vi "Main Window.vi"() -> ()   [LabVIEW 2015]
uses:
  Control Button/Exit.ctl
  Control Button/login.ctl
  Control Button/Logout.ctl
  Control Button/setting.ctl
  Control Button/report.ctl
  Control Button/Manual.ctl
  Control Button/Start.ctl
  Enqueue/Main window Seq/Test selection_1.ctl
  Enqueue/Main window Seq/Test seq_1.ctl
  Galobal variable_TI.vi
  Project Setup/Globle Variable/GR_Servo.vi
panel:
  out "Boolean 3":bool
  out "Company Name  2":string
  out "Boolean 2":bool
  out "Error 2":bool
  out "Error":bool
  out "User Name":string
  out "error out":errorcluster
  out "x = y?":bool
  out "Company Name":string
  in  "Sign In":T1
  out "Boolean":bool
  in  "Dashbord":T6
  in  "Login Window":T8 {"User Name" items=["admin", "mmum", "a", "AJAY Kumar", "", "", "", "", "", "", "", "", "", "", "", "", "", "", "", "", "", "", "", "", "", "", "", "", "", "", "", ""]}
  in  "Exit":T9
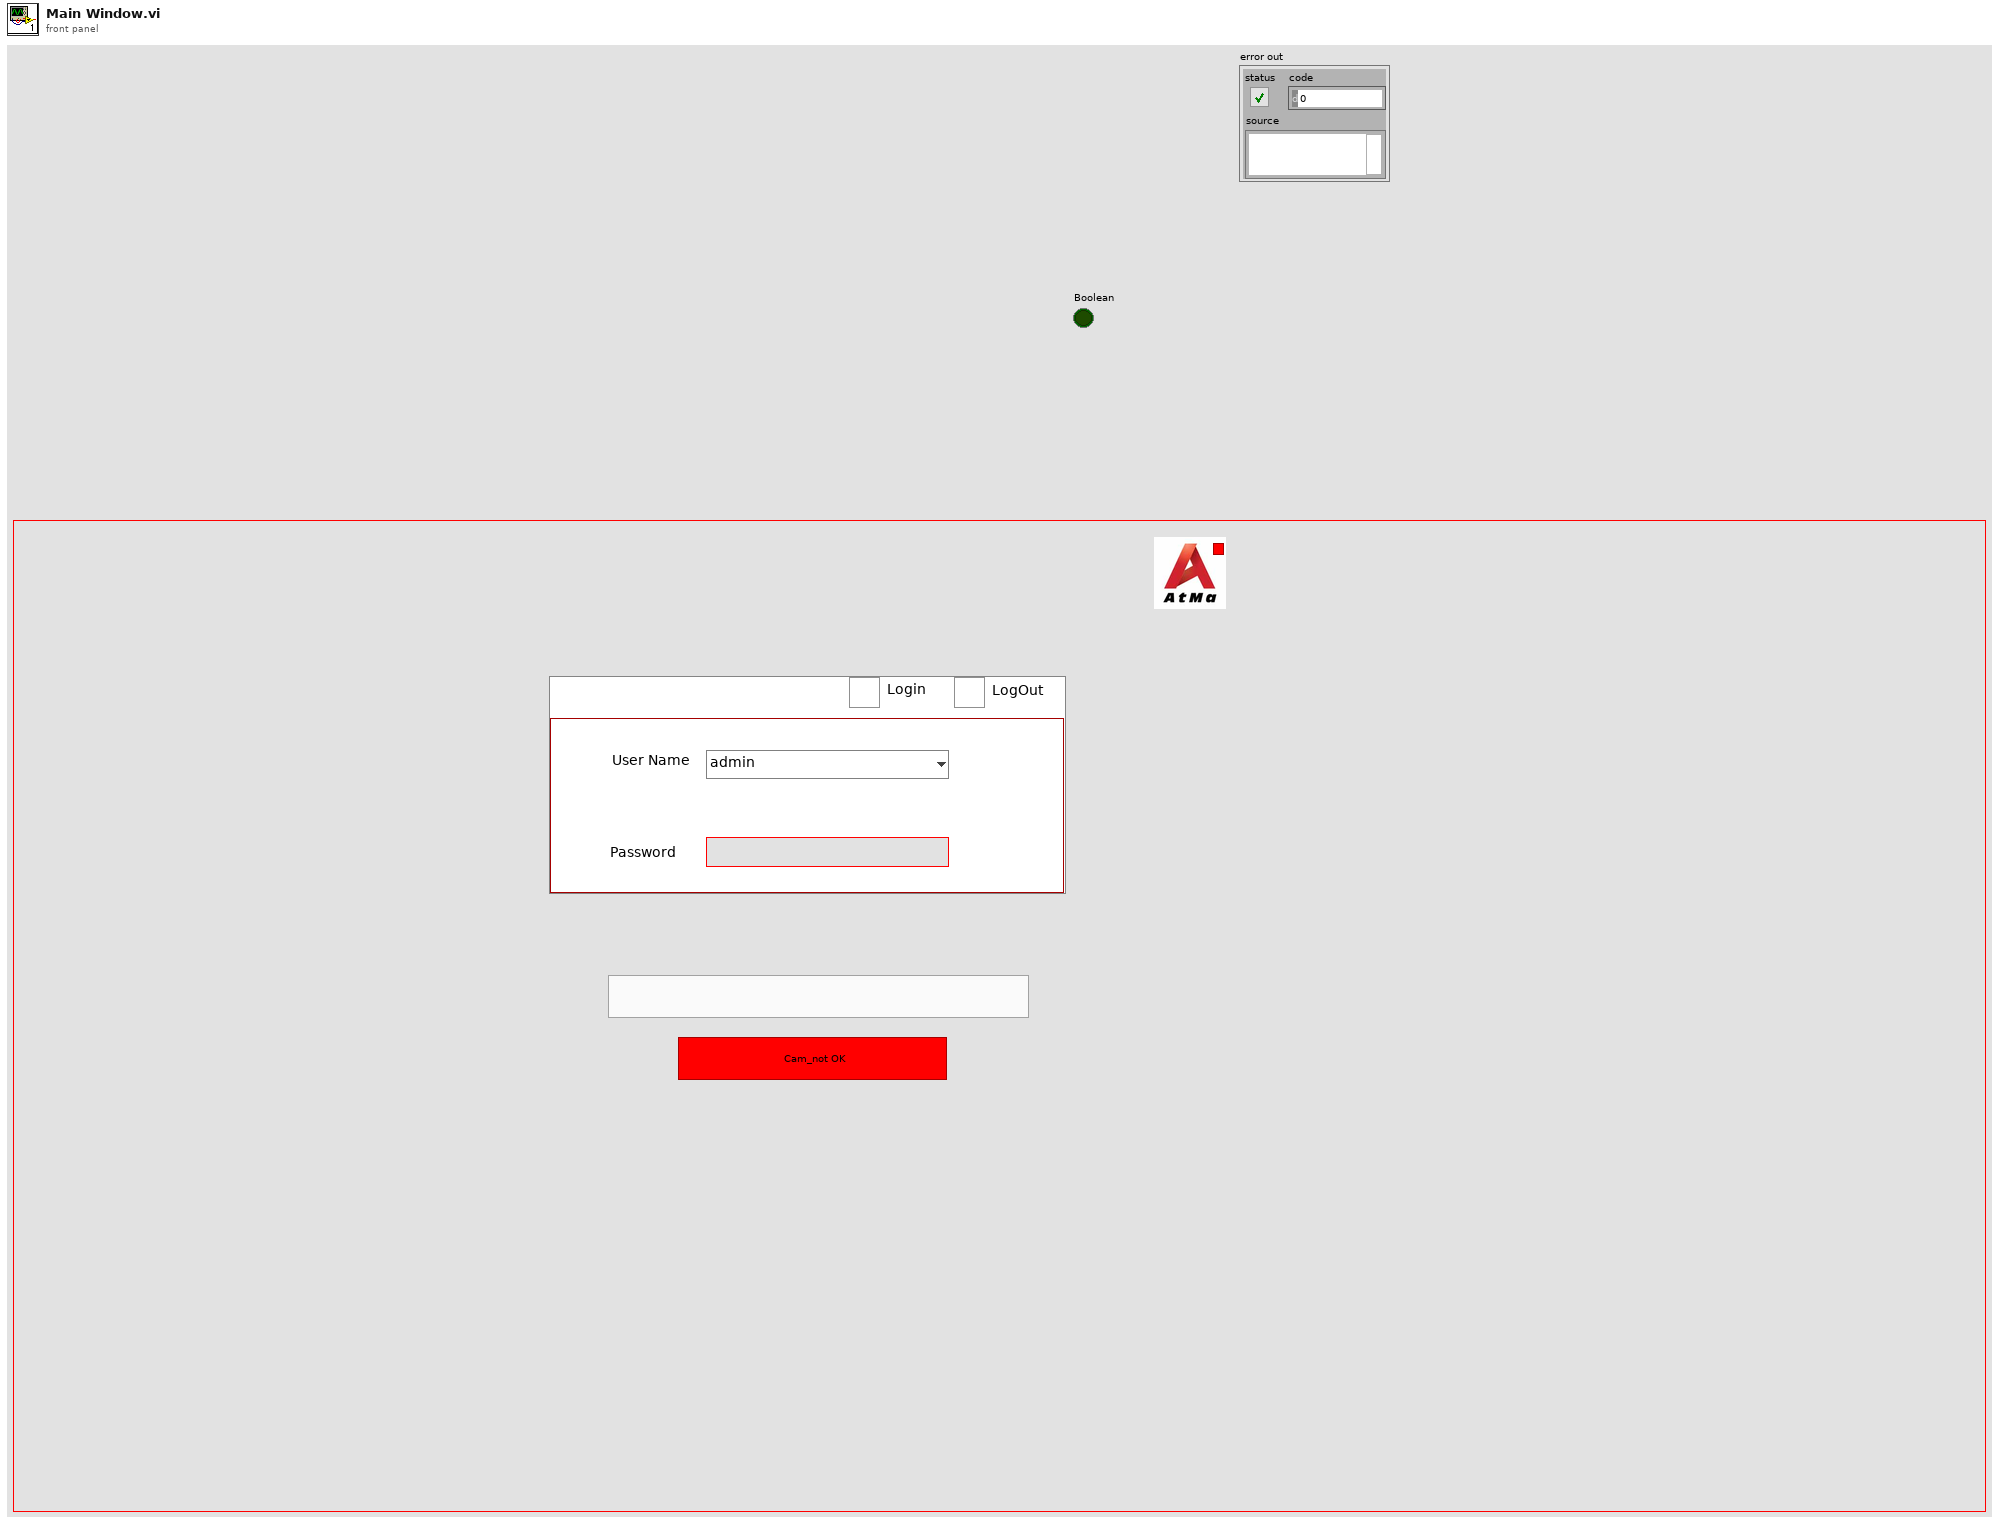
[diagram p1: front panel]
types:
  T1 = typedef "login.ctl" = bool
  T2 = typedef "setting.ctl" = bool
  T3 = typedef "report.ctl" = bool
  T4 = typedef "Manual.ctl" = bool
  T5 = typedef "Start.ctl" = bool
  T6 = cluster{"Setting":T2, "Report":T3, "Manaul":T4, "Start":T5}
  T7 = typedef "Logout.ctl" = bool
  T8 = cluster{"User Name":u16, "Password":string, "Sign In":T1, "Log Out":T7}
  T9 = typedef "Exit.ctl" = bool
  T10 = typedef "Test selection_1.ctl" = enum16{"Init", "Enqueue ", "Enqueue N", "Enqueue in stack", "Enqueue in stack N", "Dequeue", "Dequeue N", "Flush", "Release Queue"}
  T11 = typedef "Test seq_1.ctl" = enum16{"Poll Event", "Login", "Logout", "Confi", "Manual", "Report", "Testing", "Exit"}
  T12 = cluster{"XInput":dbl[], "Y New Value":dbl[], "Avg point":i16}[]
  T13 = cluster{"Slop":dbl[], "Intercept":dbl[], "Average ":i16[]}
  T14 = cluster{"UserName":string[], "Password":string[], "Usertype":string[], "Analog Min":string[], "Analog Max":string[], "DigitalInput Port":string[], "Digital Output Port":string[], "ANalog Port":string[], "IOList":cluster{"DI List_280":string[], "D0List _280":string[], "AI List_280":string[]}}
  T15 = cluster{"DI List_280":string[], "D0List _280":string[], "AI List_280":string[]}
  T16 = cluster{"DigitalInput Port[0]":string, "DigitalInput Port[1]":string, "DigitalInput Port[2]":string, "DigitalInput Port[3]":string, "DigitalInput Port[4]":string, "DigitalInput Port[5]":string, "DigitalInput Port[6]":string, "DigitalInput Port[7]":string, "DigitalInput Port[8]":string, "DigitalInput Port[9]":string, "DigitalInput Port[10]":string, "DigitalInput Port[11]":string, "DigitalInput Port[12]":string, "DigitalInput Port[13]":string, "DigitalInput Port[14]":string, "DigitalInput Port[15]":string}
  T17 = cluster{"Digital Output Port[0]":string, "Digital Output Port[1]":string, "Digital Output Port[2]":string, "Digital Output Port[3]":string, "Digital Output Port[4]":string, "Digital Output Port[5]":string, "Digital Output Port[6]":string, "Digital Output Port[7]":string, "Digital Output Port[8]":string, "Digital Output Port[9]":string, "Digital Output Port[10]":string, "Digital Output Port[11]":string, "Digital Output Port[12]":string, "Digital Output Port[13]":string, "Digital Output Port[14]":string, "Digital Output Port[15]":string, "Digital Output Port[16]":string, "Digital Output Port[17]":string, "Digital Output Port[18]":string, "Digital Output Port[19]":string, "Digital Output Port[20]":string, "Digital Output Port[21]":string, "Digital Output Port[22]":string, "Digital Output Port[23]":string, "Digital Output Port[24]":string, "Digital Output Port[25]":string}
  T18 = cluster{"ANalog Port[0]":string, "ANalog Port[1]":string, "ANalog Port[2]":string, "ANalog Port[3]":string, "ANalog Port[4]":string, "ANalog Port[5]":string, "ANalog Port[6]":string, "ANalog Port[7]":string, "ANalog Port[8]":string, "ANalog Port[9]":string, "ANalog Port[10]":string, "ANalog Port[11]":string, "ANalog Port[12]":string, "ANalog Port[13]":string, "ANalog Port[14]":string, "ANalog Port[15]":string, "ANalog Port[16]":string, "ANalog Port[17]":string, "ANalog Port[18]":string, "ANalog Port[19]":string, "ANalog Port[20]":string, "ANalog Port[21]":string, "ANalog Port[22]":string, "ANalog Port[23]":string, "ANalog Port[24]":string, "ANalog Port[25]":string, "ANalog Port[26]":string, "ANalog Port[27]":string, "ANalog Port[28]":string, "ANalog Port[29]":string, "ANalog Port[30]":string, "ANalog Port[31]":string}
  T19 = enum32{"Invalid", "Standard", "Closed", "Hidden", "Minimized", "Maximized"}
  T20 = enum8{"Enabled", "Disabled", "Disabled and Grayed Out"}
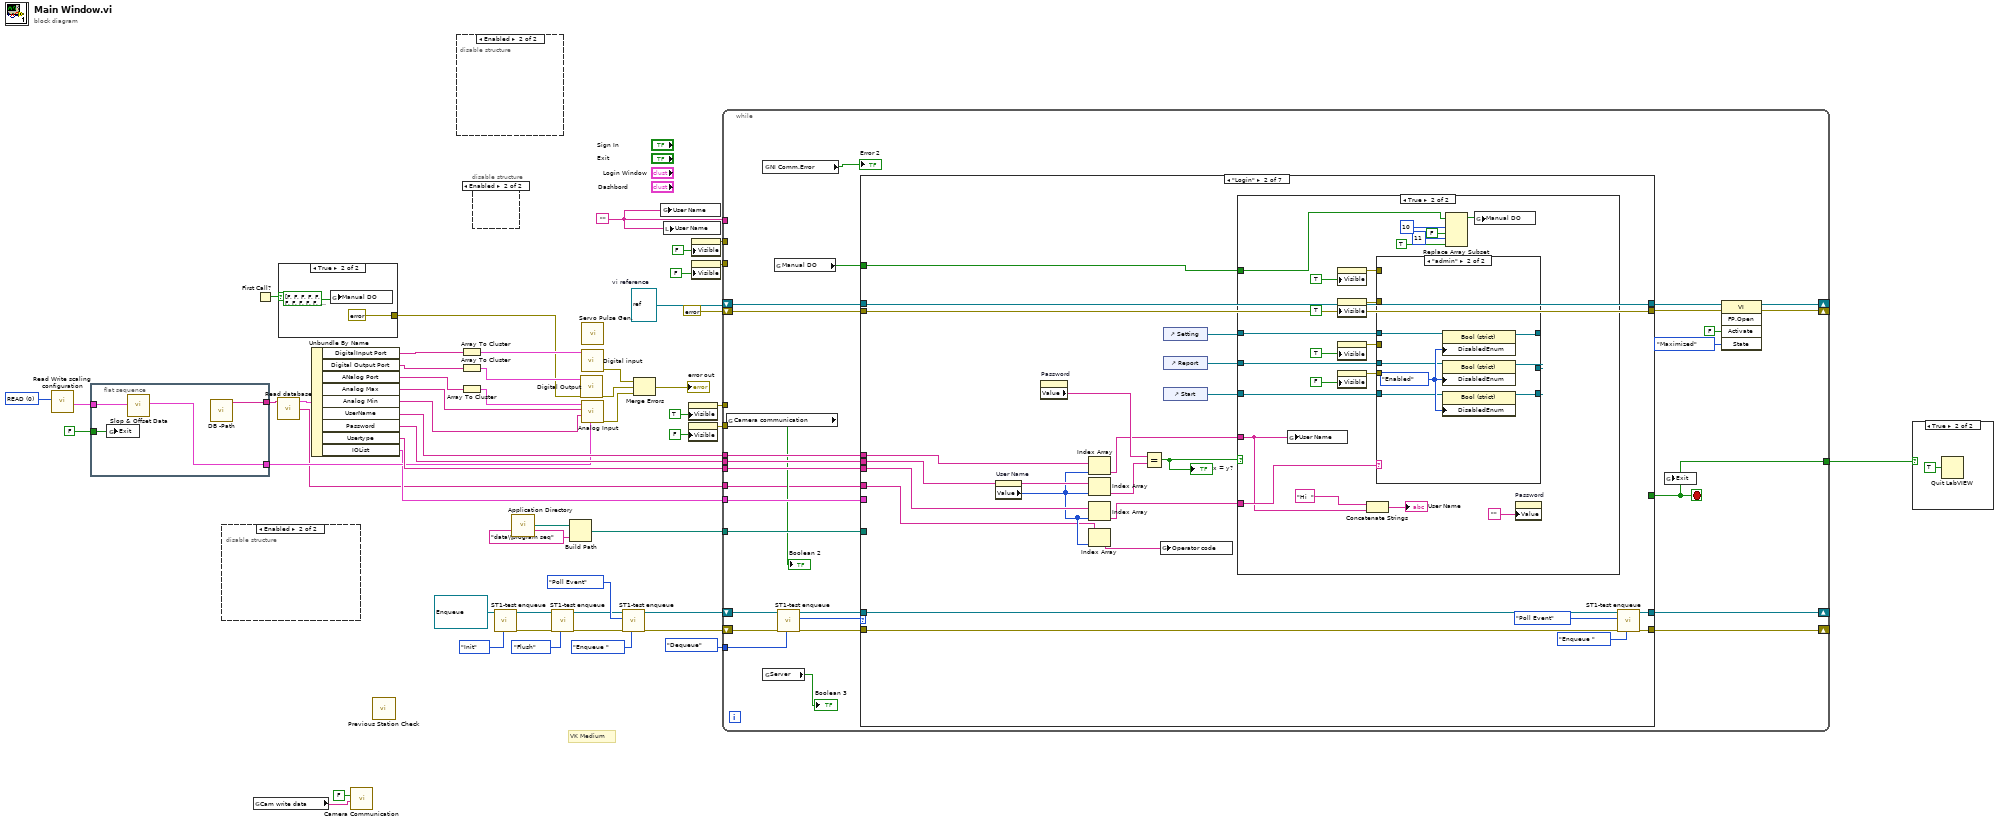
[diagram p0: block diagram]
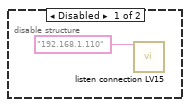
[diagram p2: hidden frame]
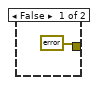
[diagram p5: hidden frame]
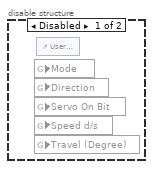
[diagram p6: hidden frame]
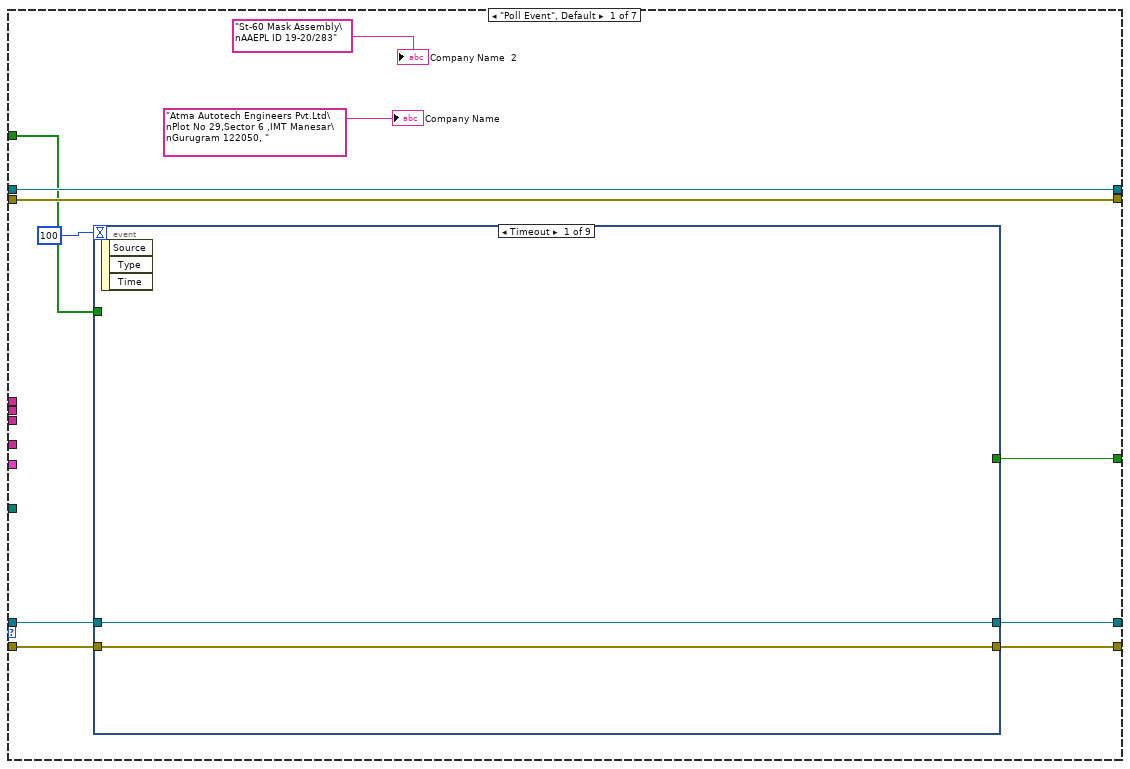
[diagram p7: hidden frame]
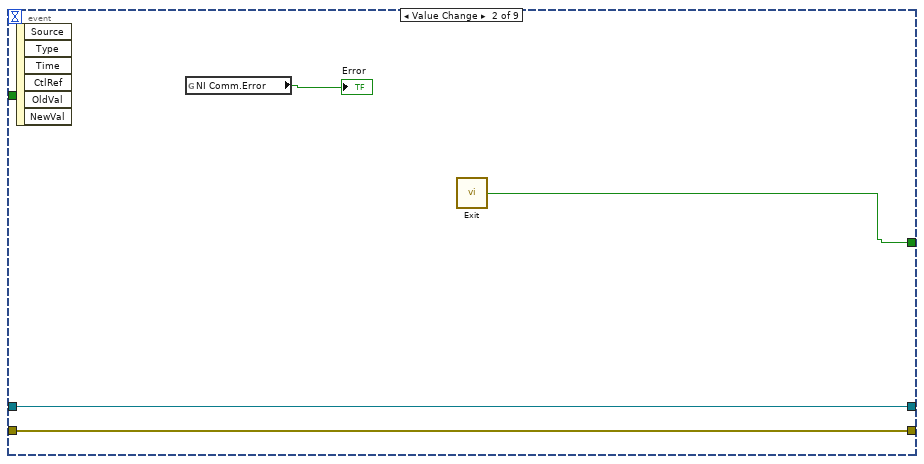
[diagram p8: hidden frame]
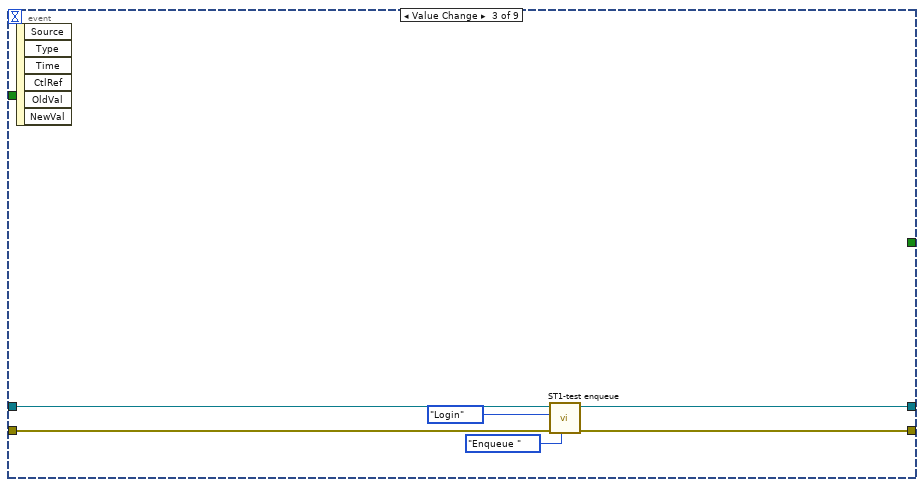
[diagram p9: hidden frame]
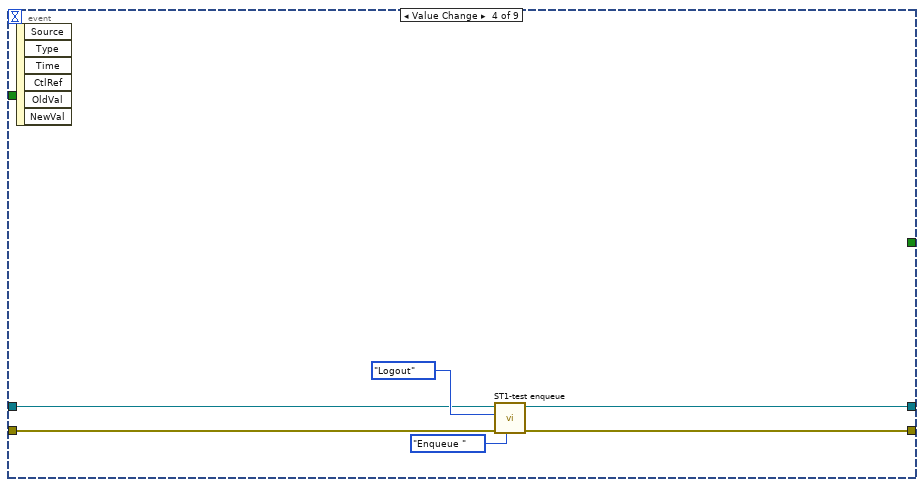
[diagram p10: hidden frame]
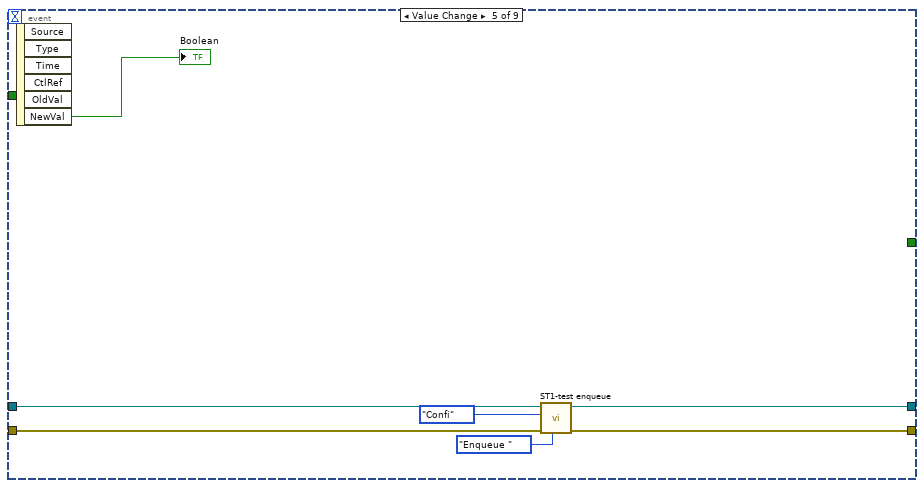
[diagram p11: hidden frame]
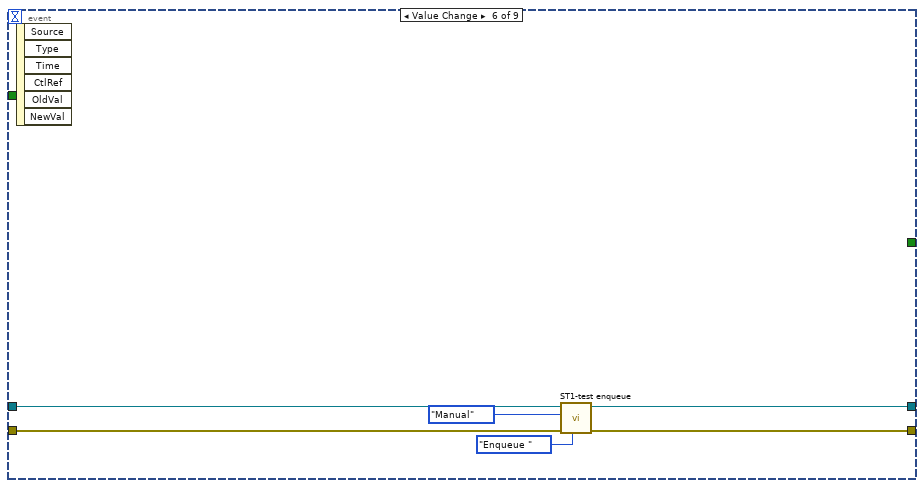
[diagram p12: hidden frame]
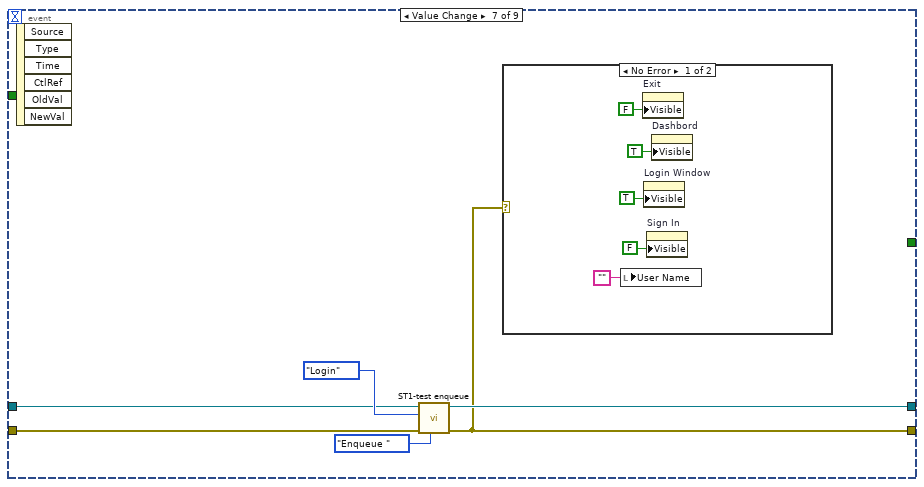
[diagram p13: hidden frame]
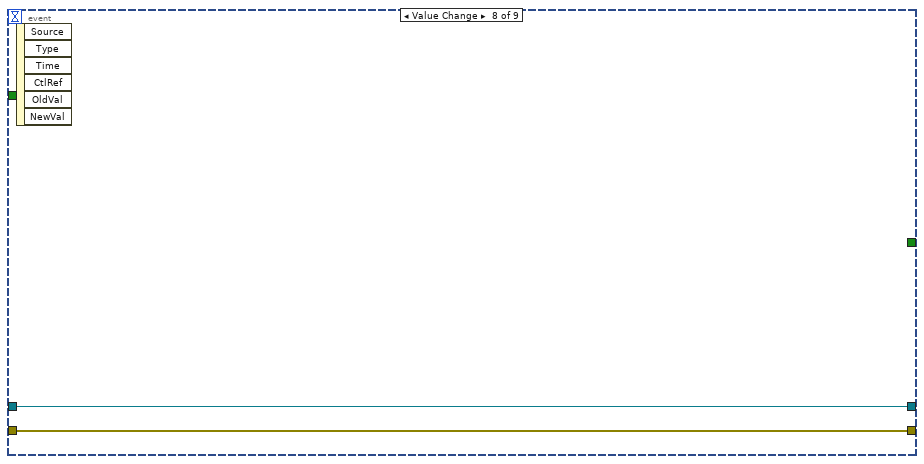
[diagram p15: hidden frame]
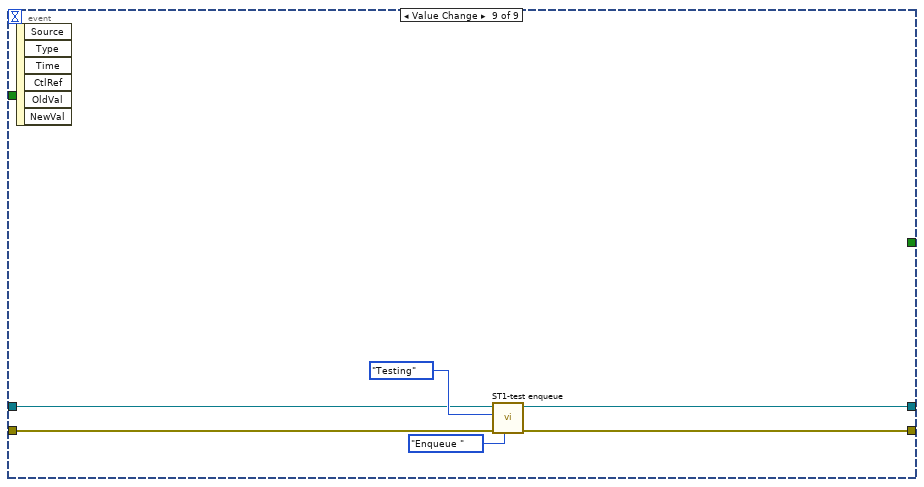
[diagram p16: hidden frame]
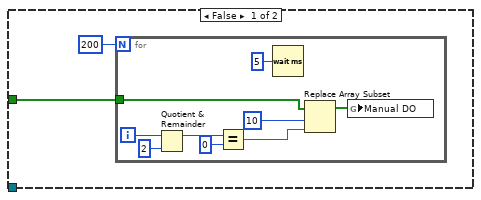
[diagram p17: hidden frame]
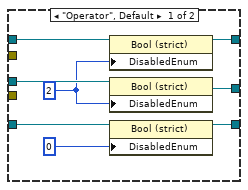
[diagram p18: hidden frame]
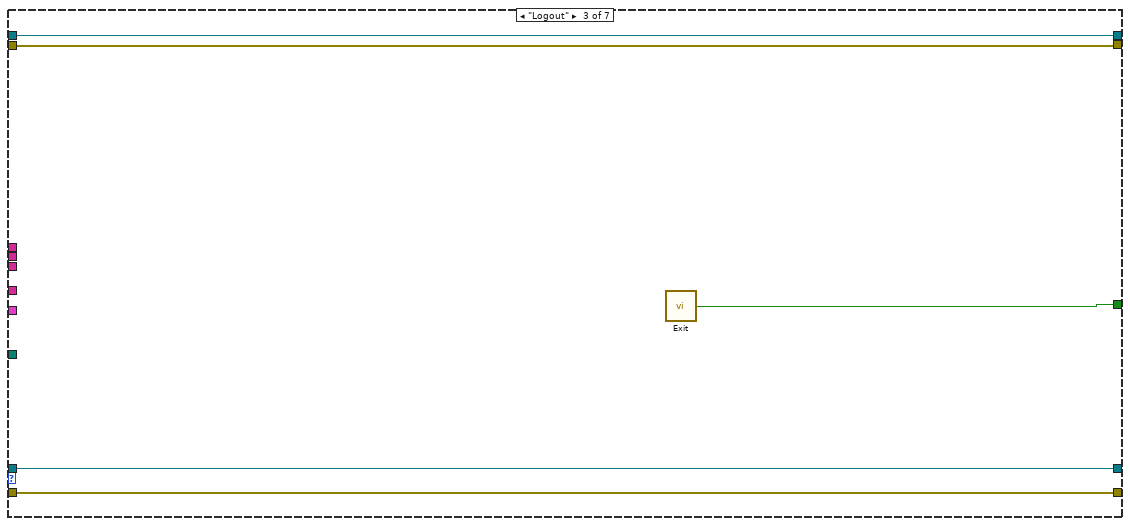
[diagram p19: hidden frame]
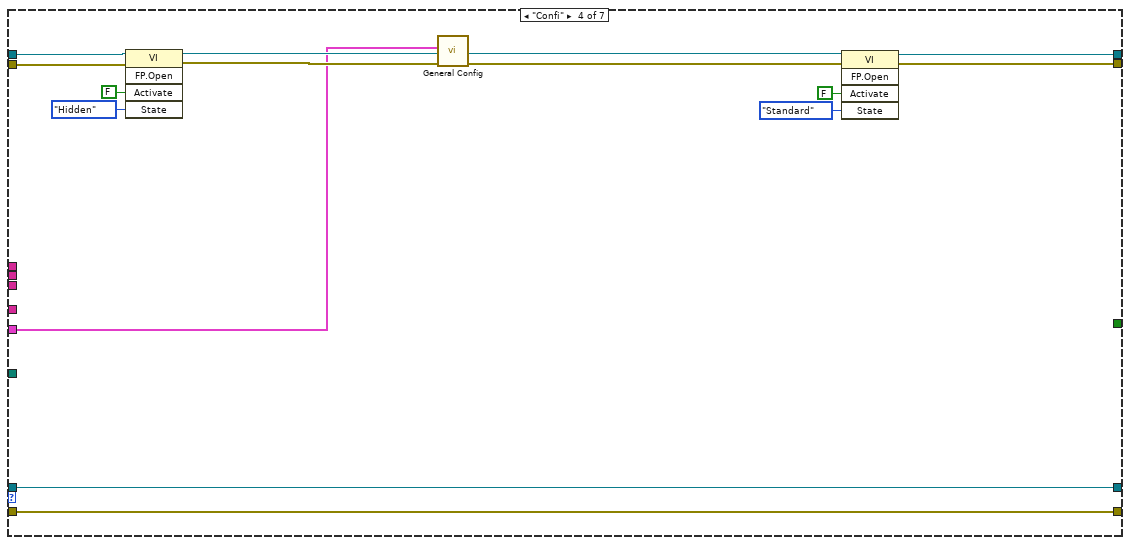
[diagram p20: hidden frame]
diagram:
  w18 = u16 0 items=["READ", "WRITE"] ("Read/Write")
  w32 = ""
  w42 = refnum<vi> refnum  # vi reference
  w43 = refnum<queue> refnum items=["Poll Event", "Login", "Logout", "Confi", "Manual", "Report", "Testing", "Exit"] ("queue in")
  # "VK Medium"
  n1 = call "Read Write scaling configuration.vi"("Read/Write"=w18) -> ("Output"=w17:T12)  [unwired: 4 in, 2 out]
  n2 = flat-sequence {
    tunnel: [w58] -> w31
    tunnel: w17 -> [w57]
    tunnel: [w56] -> w16
    tunnel: FALSE ("Exit") -> [w55]
    frame #0 {
      n3 = global write "Galobal variable_TI.vi" "Exit"(w55) -> ()
      n4 = call "Slop & Offset Data.vi"("Input"=w57) -> ("Cluster"=w56:T13)  [unwired: 10 in]
      n5 = call "DB -Path.vi"() -> ("String"=w58:string)  [unwired: 11 in]
    }
  }
  n6 = disable-structure shown="Enabled" {
    frame Disabled {
      n7 = call "listen connection LV15.vi"("service name"="192.168.1.110") -> ()  [unwired: 8 in, 2 out]
    }
    frame Enabled {
    }
  }
  n8 = global read "Galobal variable_TI.vi" "Cam write data"() -> (w2:string)
  n9 = First Call?() -> (First Call?: T/F=w7:bool)
  n10 = call "Read database.vi"("String"=w31) -> ("Operator code"=w1:string[], "DB Data"=w30:T14)  [unwired: 2 in, 1 out]
  n11 = case shown="True" w7 {
    tunnel: [errorcluster {"status"=FALSE, "code"=0, "source"=""} ("error constant") errorcluster {"status"=FALSE, "code"=0, "source"=""} ("error constant")] -> w6
    frame False {
    }
    frame True {
      n12 = global write "Galobal variable_TI.vi" "Manual DO"(bool[] [FALSE, FALSE, FALSE, FALSE, FALSE, FALSE, FALSE, FALSE, FALSE, FALSE, FALSE, FALSE, FALSE, FALSE, FALSE, FALSE, FALSE, FALSE, FALSE, FALSE, FALSE, FALSE, FALSE, FALSE, FALSE, FALSE, FALSE, FALSE, FALSE, FALSE] ("Manual DO")) -> ()
    }
  }
  n13 = Unbundle By Name(w30) -> ("DigitalInput Port"=w29:string[], "Digital Output Port"=w27:string[], "ANalog Port"=w25:string[], "Analog Max"=w23:string[], "Analog Min"=w22:string[], "UserName"=w21:string[], "Password"=w20:string[], "Usertype"=w19:string[], "IOList"=w4:T15)
  n14 = call "Camera Communication.vi"("Modle"=w2, "Trigger Cammand"=FALSE) -> ()  [unwired: 10 in]
  n15 = call "Previous Station Check.vi"() -> ()  [unwired: 12 in]
  n16 = disable-structure shown="Enabled" {
    frame Disabled {
      n17 = global read "GR_Servo.vi" "Mode"() -> ()  [unwired: 1 in]
      n18 = global read "GR_Servo.vi" "Direction"() -> ()  [unwired: 1 in]
      n19 = global read "GR_Servo.vi" "Servo On Bit"() -> ()  [unwired: 1 in]
      n20 = global read "GR_Servo.vi" "Speed d/s"() -> ()  [unwired: 1 in]
      n21 = global read "GR_Servo.vi" "Travel (Degree)"() -> ()  [unwired: 1 in]
      n22 = control-ref of="User Name"() -> ()  [unwired: 1 out]
    }
    frame Enabled {
    }
  }
  n23 = Array To Cluster(array=w29) -> (cluster=w28:T16)
  n24 = Array To Cluster(array=w27) -> (cluster=w26:T17)
  n25 = Array To Cluster(array=w25) -> (cluster=w24:T18)
  n26 = disable-structure shown="Enabled" {
    frame Disabled {
    }
    frame Enabled {
    }
  }
  n27 = call "ST1-test enqueue.vi"("Enum Selection"=Test_selection_1."Init", "queue in"=w43) -> ("error out"=w52:errorcluster, "queue Out"=w48:refnum<queue>)  [unwired: 6 in, 1 out]
  n28 = call <vilib>:"Application Directory.vi"() -> ("Application Directory"=w10:path)
  n29 = call "ST1-test enqueue.vi"("Enum Selection"=Test_selection_1."Flush", "Error In"=w52, "queue in"=w48) -> ("error out"=w50:errorcluster, "queue Out"=w47:refnum<queue>)  [unwired: 5 in, 1 out]
  n30 = Build Path(base path=w10, name or relative path="data\\program seq") -> (appended path=w8:path)
  n31 = call "Digital Output.vi"("error in"=w6, "DAQmx OutPut Setting"=w26) -> ("error out"=w14:errorcluster)  [unwired: 8 in, 1 out]
  n32 = call "Digital input.vi"("DAQmx InPut Setting"=w28) -> ("error out"=w12:errorcluster)  [unwired: 9 in, 1 out]
  n33 = call "Analog Input.vi"("clai. Parmeter"=w16, "Min Value"=w22, "Max Value"=w23, "DAQmx Analog Input Setting"=w24) -> ("error out"=w13:errorcluster)  [unwired: 6 in, 1 out]
  n34 = call "Servo Pulse Gen..vi"() -> ()  [unwired: 12 in]
  n35 = call "ST1-test enqueue.vi"("Enum Selection"=Test_selection_1."Enqueue ", "Error In"=w50, "Enqueue"=Test_seq_1."Poll Event", "queue in"=w47) -> ("error out"=w45:errorcluster, "queue Out"=w46:refnum<queue>)  [unwired: 4 in, 1 out]
  n36 = Merge Errors(w12, w14, w13) -> (→"error out":errorcluster)
  n37 = global write "Galobal variable_TI.vi" "User Name"(w32) -> ()
  n38 = local write "User Name"(w32) -> ()
  n39 = property on="Login Window" class="Clust (strict)"("Visible"=TRUE) -> (error out=w37:errorcluster)  [unwired: 2 in, 1 out]
  n40 = property on="Sign In" class="Bool (strict)"("Visible"=FALSE) -> (error out=w36:errorcluster)  [unwired: 2 in, 1 out]
  n41 = property on="Exit" class="Bool (strict)"("Visible"=FALSE) -> (error out=w34:errorcluster)  [unwired: 2 in, 1 out]
  n42 = property on="Dashbord" class="Clust (strict)"("Visible"=FALSE) -> (error out=w39:errorcluster)  [unwired: 2 in, 1 out]
  n43 = while {
    shift-right: [w83] -> _
    shift-left: w46 -> [w89]
    shift-right: [w82] -> _
    shift-left: w45 -> [w88]
    tunnel: Test_selection_1."Dequeue" ("Enum Selection") -> [w87]
    shift-right: [w74] -> _
    shift-left: errorcluster {"status"=FALSE, "code"=0, "source"=""} ("error out") -> [w80]
    shift-right: [w75] -> _
    shift-left: w42 -> [w81]
    tunnel: w39 -> [_]
    tunnel: w37 -> [_]
    tunnel: w36 -> [_]
    tunnel: w34 -> [_]
    tunnel: w32 -> [_]
    tunnel: w21 -> [w73]
    tunnel: w20 -> [w72]
    tunnel: w19 -> [w71]
    tunnel: w4 -> [w70]
    tunnel: w8 -> [w69]
    tunnel: [w67] -> w5
    tunnel: w1 -> [w63]
    stop <- w67 stop-if-true
    n44 = global read "Galobal variable_TI.vi" "Camera communication"() -> (→"Boolean 2":bool)
    n45 = global read "Galobal variable_TI.vi" "NI Comm.Error"() -> (→"Error 2":bool)
    n46 = global read "Galobal variable_TI.vi" "Server"() -> (→"Boolean 3":bool)
    n47 = global read "Galobal variable_TI.vi" "Manual DO"() -> (w68:bool[])
    n48 = call "ST1-test enqueue.vi"("Enum Selection"=w87, "Error In"=w88, "queue in"=w89) -> ("error out"=w84:errorcluster, "D-enqueue"=w86:T11, "queue Out"=w85:refnum<queue>)  [unwired: 5 in]
    n49 = case shown="\"Login\"" w86 {
      tunnel: [w98 _ w222 _ _ _ _] -> w67
      tunnel: w85 -> [w99 w155 w226 w240 w248 w258 w275]
      tunnel: w84 -> [w100 w154 w225 w239 w247 w257 w274]
      tunnel: [w97 w158 w226 w240 w248 w258 w275] -> w83
      tunnel: [w96 w157 w225 w239 w247 w257 w274] -> w82
      tunnel: [w95 w167 w224 w234 w243 w256 w261] -> w77
      tunnel: [w94 w166 w223 w233 w244 w254 w259] -> w76
      tunnel: w81 -> [w95 w167 w224 w232 w245 w256 w267]
      tunnel: w80 -> [w94 w166 w223 w231 w246 w255 w270]
      tunnel: w73 -> [_ w164 _ _ _ _ _]
      tunnel: w72 -> [_ w163 _ _ _ _ _]
      tunnel: w71 -> [_ w162 _ _ _ _ _]
      tunnel: w70 -> [_ _ _ w227 w242 _ w273]
      tunnel: w69 -> [_ _ _ _ _ _ w265]
      tunnel: w68 -> [w91 w156 _ _ _ _ _]
      tunnel: w63 -> [_ w152 _ _ _ _ _]
      frame "Poll Event", Default {
        n50 = event shown="[0] Timeout" {
          selector: _ -> [_ _ _ _ _ _ _ _ _]
          dyn-events: _ -> [_ _ _ _ _ _ _ _ _]
          timeout: 100 -> [_ _ _ _ _ _ _ _ _]
          tunnel: [_ w104 _ _ _ _ _ _ _] -> w98
          tunnel: w100 -> [w101 w105 w110 w113 w121 w129 w135 w143 w147]
          tunnel: w99 -> [w102 w106 w111 w114 w122 w127 w134 w144 w148]
          tunnel: [w102 w106 w109 w116 w120 w126 w133 w144 w146] -> w97
          tunnel: [w101 w105 w108 w115 w119 w128 w132 w143 w145] -> w96
          tunnel: w91 -> [_ _ _ _ _ _ _ _ _]
          event Timeout {
            n51 = event-data() -> ()  [unwired: 1 in, 3 out]
          }
          event Value Change {
            n52 = event-data() -> ()  [unwired: 1 in, 6 out]
            n53 = global read "Galobal variable_TI.vi" "NI Comm.Error"() -> (→"Error":bool)
            n54 = call "Exit.vi"() -> ("Exit"=w104:bool)  [unwired: 1 in]
          }
          event Value Change {
            n55 = event-data() -> ()  [unwired: 1 in, 6 out]
            n56 = call "ST1-test enqueue.vi"("Enum Selection"=Test_selection_1."Enqueue ", "Error In"=w110, "Enqueue"=Test_seq_1."Login", "queue in"=w111) -> ("error out"=w108:errorcluster, "queue Out"=w109:refnum<queue>)  [unwired: 4 in, 1 out]
          }
          event Value Change {
            n57 = event-data() -> ()  [unwired: 1 in, 6 out]
            n58 = call "ST1-test enqueue.vi"("Enum Selection"=Test_selection_1."Enqueue ", "Error In"=w113, "Enqueue"=Test_seq_1."Logout", "queue in"=w114) -> ("error out"=w115:errorcluster, "queue Out"=w116:refnum<queue>)  [unwired: 4 in, 1 out]
          }
          event Value Change {
            n59 = event-data() -> ("NewVal"=→"Boolean":T2)  [unwired: 1 in, 5 out]
            n60 = call "ST1-test enqueue.vi"("Enum Selection"=Test_selection_1."Enqueue ", "Error In"=w121, "Enqueue"=Test_seq_1."Confi", "queue in"=w122) -> ("error out"=w119:errorcluster, "queue Out"=w120:refnum<queue>)  [unwired: 4 in, 1 out]
          }
          event Value Change {
            n61 = event-data() -> ()  [unwired: 1 in, 6 out]
            n62 = call "ST1-test enqueue.vi"("Enum Selection"=Test_selection_1."Enqueue ", "Error In"=w129, "Enqueue"=Test_seq_1."Manual", "queue in"=w127) -> ("error out"=w128:errorcluster, "queue Out"=w126:refnum<queue>)  [unwired: 4 in, 1 out]
          }
          event Value Change {
            n63 = event-data() -> ()  [unwired: 1 in, 6 out]
            n64 = call "ST1-test enqueue.vi"("Enum Selection"=Test_selection_1."Enqueue ", "Error In"=w135, "Enqueue"=Test_seq_1."Login", "queue in"=w134) -> ("error out"=w132:errorcluster, "queue Out"=w133:refnum<queue>)  [unwired: 4 in, 1 out]
            n65 = case shown="No Error" w132 {
              frame No Error {
                n66 = local write "User Name"("") -> ()
                n67 = property on="Exit" class="Bool (strict)"("Visible"=FALSE) -> ()  [unwired: 2 in, 2 out]
                n68 = property on="Login Window" class="Clust (strict)"("Visible"=TRUE) -> ()  [unwired: 2 in, 2 out]
                n69 = property on="Sign In" class="Bool (strict)"("Visible"=FALSE) -> ()  [unwired: 2 in, 2 out]
                n70 = property on="Dashbord" class="Clust (strict)"("Visible"=TRUE) -> ()  [unwired: 2 in, 2 out]
              }
              frame Error {
              }
            }
          }
          event Value Change {
            n71 = event-data() -> ()  [unwired: 1 in, 6 out]
          }
          event Value Change {
            n72 = event-data() -> ()  [unwired: 1 in, 6 out]
            n73 = call "ST1-test enqueue.vi"("Enum Selection"=Test_selection_1."Enqueue ", "Error In"=w147, "Enqueue"=Test_seq_1."Testing", "queue in"=w148) -> ("error out"=w145:errorcluster, "queue Out"=w146:refnum<queue>)  [unwired: 4 in, 1 out]
          }
        }
        "Company Name" <- "Atma Autotech Engineers Pvt.Ltd\nPlot No 29,Sector 6 ,IMT Manesar\nGurugram 122050, " ("string")
        "Company Name  2" <- "St-60 Mask Assembly\nAAEPL ID 19-20/283" ("string")
      }
      frame "Login" {
        n74 = property on="User Name" class="Ring (strict)"() -> ("Value"=w153:u16)  [unwired: 2 in, 2 out]
        n75 = property on="Password" class="Str"() -> ("Value"=w172:string)  [unwired: 2 in, 2 out]
        n76 = Index Array(array=w152, index=w153) -> (element=w151:string)
        n77 = Index Array(array=w164, index=w153) -> (element=w165:string)
        n78 = Index Array(array=w163, index=w153) -> (element=w173:string)
        n79 = Index Array(array=w162, index=w153) -> (element=w171:string)
        n80 = Equal?(x=w172, y=w173) -> (x = y?=w161:bool)
        "x = y?" <- w161
        n81 = global write "Galobal variable_TI.vi" "Operator code"(w151) -> ()
        n82 = control-ref of="Setting"() -> (w170:refnum<vi>)
        n83 = control-ref of="Report"() -> (w168:refnum<vi>)
        n84 = control-ref of="Start"() -> (w169:refnum<vi>)
        n85 = case shown="True" w161 {
          tunnel: w171 -> [_ w202]
          tunnel: w170 -> [_ w206]
          tunnel: w168 -> [_ w205]
          tunnel: w169 -> [_ w204]
          tunnel: w165 -> [_ w185]
          tunnel: w156 -> [w174 w189]
          frame False {
            n86 = for {
              N: 200 -> [_]
              tunnel: w174 -> [w176]
              i -> [w184]
              n87 = Quotient & Remainder(x=w184, y=2) -> (x-y*floor(x/y)=w182:i32)  [unwired: 1 out]
              n88 = Equal?(x=w182, y=0) -> (x = y?=w179:bool)
              n89 = Wait (ms)(milliseconds to wait=u32 5) -> ()  [unwired: 1 out]
              n90 = Replace Array Subset(array=w176, new element=w179, index=10) -> (w177:bool[])
              n91 = global write "Galobal variable_TI.vi" "Manual DO"(w177) -> ()
            }
          }
          frame True {
            n92 = global write "Galobal variable_TI.vi" "User Name"(w185) -> ()
            n93 = property on="Exit" class="Bool (strict)"("Visible"=TRUE) -> (error out=w193:errorcluster)  [unwired: 2 in, 1 out]
            n94 = property on="Dashbord" class="Clust (strict)"("Visible"=TRUE) -> (error out=w198:errorcluster)  [unwired: 2 in, 1 out]
            n95 = property on="Sign In" class="Bool (strict)"("Visible"=TRUE) -> (error out=w197:errorcluster)  [unwired: 2 in, 1 out]
            n96 = property on="Login Window" class="Clust (strict)"("Visible"=FALSE) -> (error out=w199:errorcluster)  [unwired: 2 in, 1 out]
            n97 = Concatenate Strings("Hi  " ("string"), w185) -> (→"User Name":string)
            n98 = case shown="\"admin\"" w202 {
              tunnel: [w214 w220] -> _
              tunnel: [w213 w219] -> _
              tunnel: [w212 w218] -> _
              tunnel: w206 -> [w211 w217]
              tunnel: w205 -> [w210 w216]
              tunnel: w204 -> [w209 w215]
              tunnel: w199 -> [_ _]
              tunnel: w198 -> [_ _]
              tunnel: w197 -> [_ _]
              tunnel: w193 -> [_ _]
              frame "Operator", Default {
                w207 = 2
                n99 = property class="Bool (strict)"(reference=w211, "DisabledEnum"=w207) -> (reference out=w214:refnum<vi>)  [unwired: 1 in, 1 out]
                n100 = property class="Bool (strict)"(reference=w210, "DisabledEnum"=w207) -> (reference out=w213:refnum<vi>)  [unwired: 1 in, 1 out]
                n101 = property class="Bool (strict)"(reference=w209, "DisabledEnum"=0) -> (reference out=w212:refnum<vi>)  [unwired: 1 in, 1 out]
              }
              frame "admin" {
                w221 = T20."Enabled" ("Disabled")
                n102 = property class="Bool (strict)"(reference=w217, "DisabledEnum"=w221) -> (reference out=w220:refnum<vi>)  [unwired: 1 in, 1 out]
                n103 = property class="Bool (strict)"(reference=w216, "DisabledEnum"=w221) -> (reference out=w219:refnum<vi>)  [unwired: 1 in, 1 out]
                n104 = property class="Bool (strict)"(reference=w215, "DisabledEnum"=w221) -> (reference out=w218:refnum<vi>)  [unwired: 1 in, 1 out]
              }
            }
            n105 = Replace Array Subset(array=w189, new element #1=FALSE ("new element/subarray"), index #1=10 ("index"), new element #2=TRUE ("new element/subarray"), index #2=11 ("index")) -> (w190:bool[])
            n106 = global write "Galobal variable_TI.vi" "Manual DO"(w190) -> ()
            n107 = property on="Password" class="Str"("Value"="") -> ()  [unwired: 2 in, 2 out]
          }
        }
        n108 = call "ST1-test enqueue.vi"("Enum Selection"=Test_selection_1."Enqueue ", "Error In"=w154, "Enqueue"=Test_seq_1."Poll Event", "queue in"=w155) -> ("error out"=w157:errorcluster, "queue Out"=w158:refnum<queue>)  [unwired: 4 in, 1 out]
      }
      frame "Logout" {
        n109 = call "Exit.vi"() -> ("Exit"=w222:bool)  [unwired: 1 in]
      }
      frame "Confi" {
        n110 = invoke class="VI" method="FP.Open"(reference=w232, error in=w231, "Activate"=FALSE ("Activate?"), "State"=T19."Hidden") -> (reference out=w228:refnum<vi>, error out=w230:errorcluster)  [unwired: 1 in, 3 out]
        n111 = call "General Config.vi"("error In"=w230, "IOList"=w227) -> ("error out"=w229:errorcluster)  [unwired: 8 in, 1 out]
        n112 = invoke class="VI" method="FP.Open"(reference=w228, error in=w229, "Activate"=FALSE ("Activate?"), "State"=T19."Standard") -> (reference out=w234:refnum<vi>, error out=w233:errorcluster)  [unwired: 1 in, 3 out]
      }
      frame "Manual" {
        w241 = TRUE ("Manual CMD")
        n113 = global write "Galobal variable_TI.vi" "Manual CMD"(w241) -> ()
        n114 = flat-sequence {
          tunnel: w246 -> [w253]
          tunnel: w245 -> [w252]
          tunnel: [w251] -> w244
          tunnel: [w250] -> w243
          tunnel: w242 -> [w249]
          tunnel: w241 -> [_]
          frame #0 {
            n115 = call "Manual.vi"("vi reference"=w252, "error in (no error)"=w253, "IOList_280"=w249) -> ("error out"=w251:errorcluster, "Out reference"=w250:refnum<vi>)  [unwired: 7 in]
          }
        }
      }
      frame "Report" {
        n116 = call "Report read csv G.vi"("error in"=w255) -> ("error out"=w254:errorcluster)  [unwired: 2 in]
      }
      frame "Testing" {
        n117 = Unbundle By Name(w273) -> ("DI List_280"=w266:string[])
        n118 = invoke class="VI" method="FP.Open"(reference=w267, error in=w270, "Activate"=FALSE ("Activate?"), "State"=T19."Hidden") -> (reference out=w269:refnum<vi>, error out=w268:errorcluster)  [unwired: 1 in, 3 out]
        n119 = call "Program list Selection.vi"("error in"=w268, "FeedBack Channel"=w266, "Filepath"=w265, "vi referenceIn"=w269) -> ("error out"=w260:errorcluster, "vi reference Out"=w262:refnum<vi>)  [unwired: 4 in, 2 out]
        n120 = invoke class="VI" method="FP.Open"(reference=w262, error in=w260, "Activate"=FALSE ("Activate?"), "State"=T19."Standard") -> (reference out=w261:refnum<vi>, error out=w259:errorcluster)  [unwired: 1 in, 3 out]
      }
    }
    n121 = global write "Galobal variable_TI.vi" "Exit"(w67) -> ()
    n122 = invoke class="VI" method="FP.Open"(reference=w77, error in=w76, "Activate"=FALSE ("Activate?"), "State"=T19."Maximized") -> (reference out=w75:refnum<vi>, error out=w74:errorcluster)  [unwired: 1 in, 3 out]
  }
  n123 = case shown="True" w5 {
    frame False {
    }
    frame True {
      n124 = Quit LabVIEW(quit? (T)=TRUE) -> ()
    }
  }
